vi "Send Data API.vi"(8 "Error In":errorcluster, 10 "Data DVR":refnum<data-value>, 11 "Type DVR":refnum<data-value>) -> (0 "Error Out":errorcluster, 3 "Type DVR Out":refnum<data-value>)   [LabVIEW 2020, in "Communication.lvclass"]
doc: "The method is a API that accepts the DVR of the communication class and data class to perform the over riding method to send data."
uses:
  Communication.lvclass
  Data/Data.lvclass
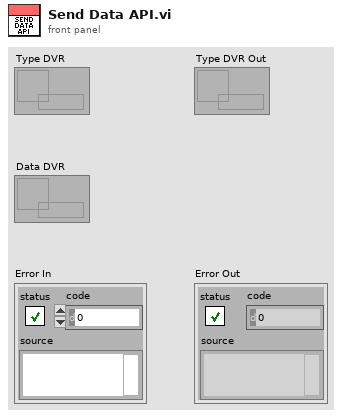
[diagram p1: front panel]
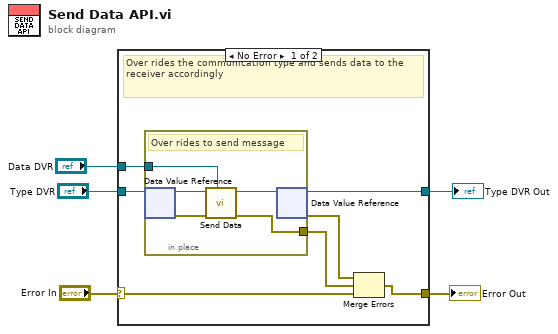
[diagram p0: block diagram]
diagram:
  n1 = case shown="No Error" "Error In" {
    selector: "Error In" -> [w12 w19]
    tunnel: [w8 w19] -> w4
    tunnel: "Type DVR" -> [w11 w18]
    tunnel: "Data DVR" -> [w10 _]
    tunnel: [w9 w18] -> w1
    frame No Error {
      # "Over rides the communication type and sends data to the receiver accordingly"
      n2 = in-place {
        in-place-border: [w16] -> w7
        in-place-border: w10 -> [w13]
        # "Over rides to send message"
        n3 = in-place-dvr #1(w11) -> (w15:refnum<class "Communication.lvclass">, w17:errorcluster)
        n4 = call-dynamic "Send Data.vi"("Data DVR"=w13, "Error In"=w17, "Communication in"=w15) -> ("Error Out"=w16:errorcluster, "Communication out"=w14:refnum<class "Communication.lvclass">)  [unwired: 7 in]
        n5 = in-place-dvr #1(w14) -> (w9:refnum<data-value>, w6:errorcluster)
      }
      n6 = Merge Errors(w6, w7, w12) -> (w8:errorcluster)
    }
    frame Error {
    }
  }
  "Error Out" <- w4
  "Type DVR Out" <- w1
